vi "PID Angle Testing.vi"() -> ()   [LabVIEW 2016]
uses:
  <vilib>/Rock Robotics/WPI/Utilities/WPI_GetSetVariantRefNum.vi
  <vilib>/addons/control/pid/pid.llb/PID (DBL).vi
  <vilib>/Rock Robotics/WPI/RobotDrive/WPI_RobotDriveArcadeDrive_Standard(NoSaturation).vi
  <vilib>/addons/control/pid/NI_PID_pid.lvlib
panel:
  in  "Angle":bool=TRUE
  in  "Reset Gyro":bool
  in  "angle A":dbl
  in  "angle B":dbl=90.0
  out "Waveform Chart":cluster{"f":dbl, dbl}(graph)
  in  "Chart slowing":i32(knob)=1 scale=1.0..10.0
  in  "Angle Gains":T1={"proportional gain (Kc)"=0.01, "integral time (Ti, min)"=0.0, "derivative time (Td, min)"=0.0}
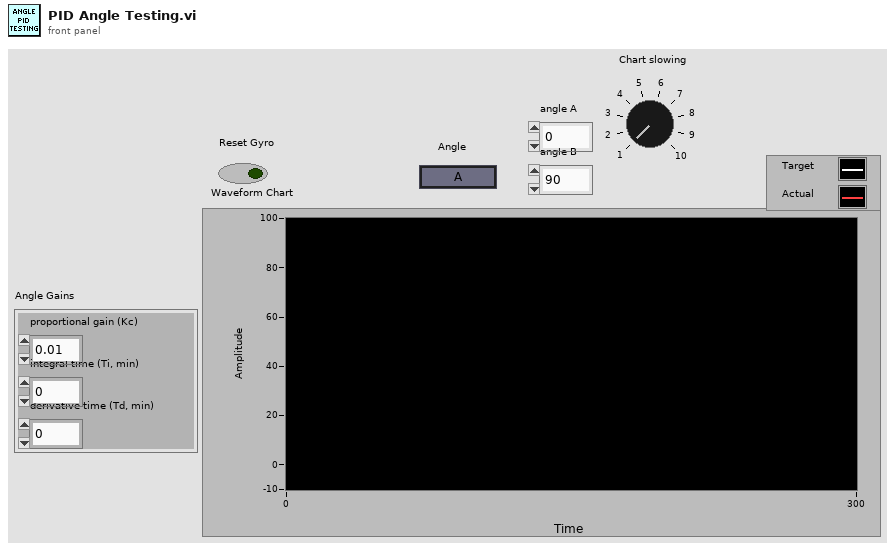
[diagram p1: front panel]
types:
  T1 = cluster{"proportional gain (Kc)":dbl, "integral time (Ti, min)":dbl, "derivative time (Td, min)":dbl}
  T2 = typedef "WPI_RobotDriveDevRef.ctl" = cluster{"DevStatus":errorcluster, "Motors[]":T3[], "Square Inputs":bool, "Max Output":dbl}
  T3 = typedef "WPI_MotorControlDeviceRef.ctl" = cluster{"DeviceStatus":errorcluster, "Type":T4, "PWM":cluster{"PWM Channel":T5, "DeadBand":T6}, "CAN":cluster{"Device Number":u8, "SetOutput VI Ref":variant, "GetOutput VI Ref":variant, "Enable VI Ref":variant, "Disable VI Ref":variant, "Data":variant}, "Invert":bool}
  T4 = typedef "WPI_MotorControlType.ctl" = enum16{"PWM", "CAN"}
  T5 = typedef "FPGA_DIOPWMChannel.ctl" = enum8{"PWM 0", "PWM 1", "PWM 2", "PWM 3", "PWM 4", "PWM 5", "PWM 6", "PWM 7", "PWM 8", "PWM 9", "PWM MXP 0", "PWM MXP 1", "PWM MXP 2", "PWM MXP 3", "PWM MXP 4", "PWM MXP 5", "PWM MXP 6", "PWM MXP 7", "PWM MXP 8", "PWM MXP 9", "Invalid"}
  T6 = typedef "WPI_PWMDeadband.ctl" = cluster{"Name":string, "maxPositivePwm":i32, "minPositivePwm":i32, "centerPwm":i32, "maxNegativePwm":i32, "minNegativePwm":i32, "angularRange":u16}
  T7 = cluster{"Yaw":dbl, "Roll":dbl, "Pitch":dbl, "Heading":dbl, "Fused Heading":dbl}
  T8 = cluster{"proportional gain (Kc)":dbl, "f":dbl, "derivative time (Td, min)":dbl}
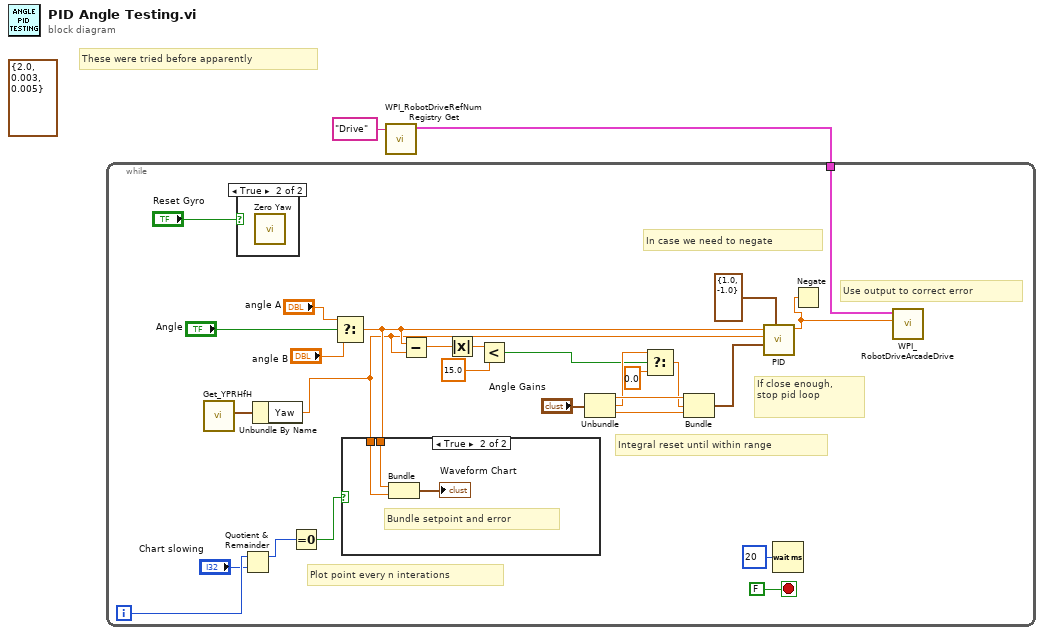
[diagram p0: block diagram]
diagram:
  (unwired) T1 {"proportional gain (Kc)"=2.0, "integral time (Ti, min)"=0.003, "derivative time (Td, min)"=0.005} ("Drive straight")
  # "These were tried before apparently"
  n1 = call <vilib>:"WPI_RobotDriveRefNum Registry Get.vi"("refnum name"="Drive") -> ("RobotDriveDevRef"=w1:T2)  [unwired: 9 in, 1 out]
  n2 = while {
    tunnel: w1 -> [w20]
    i -> [w22]
    stop <- FALSE stop-if-true
    # "Integral reset until within range"
    # "In case we need to negate"
    # "Plot point every n interations"
    # "If close enough,\nstop pid loop"
    # "Use output to correct error"
    n3 = call <vilib>:"Get_YPRHfH.vi"() -> ("YRPHfH"=w17:T7)  [unwired: 11 in]
    n4 = case shown="True" "Reset Gyro" {
      frame False {
      }
      frame True {
        n5 = call <vilib>:"Zero Yaw.vi"() -> ()  [unwired: 12 in]
      }
    }
    n6 = Quotient & Remainder(x=w22, y="Chart slowing") -> (x-y*floor(x/y)=w24:i32)  [unwired: 1 out]
    n7 = Unbundle By Name(w17) -> ("Yaw"=w11:dbl)
    n8 = Equal To 0?(x=w24) -> (x = 0?=w23:bool)
    n9 = Select(t="angle A", s="Angle", f="angle B") -> (s? t:f=w12:dbl)
    n10 = case shown="True" w23 {
      tunnel: w12 -> [_ w31]
      tunnel: w11 -> [_ w30]
      frame False {
      }
      frame True {
        # "Bundle setpoint and error"
        n11 = Bundle("angle B"=w31, "Yaw"=w30) -> (→"Waveform Chart":cluster{"angle B":dbl, "Yaw":dbl})  [unwired: 1 in]
      }
    }
    n12 = Subtract(x=w12, y=w11) -> (x-y=w10:dbl)
    n13 = Absolute Value(x=w10) -> (abs(x)=w15:dbl)
    n14 = Less?(x=w15, y=15.0) -> (x < y?=w5:bool)
    n15 = Unbundle("Angle Gains") -> ("proportional gain (Kc)"=w9:dbl, "integral time (Ti, min)"=w6:dbl, "derivative time (Td, min)"=w8:dbl)
    n16 = Select(t=w6, s=w5, f=0.0) -> (s? t:f=w3:dbl)
    n17 = Bundle("proportional gain (Kc)"=w9, "f"=w3, "derivative time (Td, min)"=w8) -> (w7:T8)  [unwired: 1 in]
    n18 = call-poly <vilib>:"PID.vi"("output range"=cluster{"output high":dbl, "output low":dbl} {"output high"=1.0, "output low"=-1.0}, "PID gains"=w7, "process variable"=w11, "setpoint"=w12) -> ("output"=w19:dbl)  [unwired: 6 in, 1 out]
    n19 = Wait (ms)(milliseconds to wait=u32 20) -> ()  [unwired: 1 out]
    n20 = Negate(x=w19) -> ()  [unwired: 1 out]
    n21 = call-poly <vilib>:"WPI_RobotDriveArcadeDrive.vi"("X axis value"=w19, "RobotDriveDevRef"=w20) -> ()  [unwired: 7 in, 3 out]
  }
